vi "LabVIEW MakerHub Speed Direction State Machine.vi"() -> ()   [LabVIEW 2011]
panel:
  out "Speed Chart":dbl(graph)
  in  "Idle":bool
  out "State":T1(ring)=enum."fullreverse"
  in  "Max Speed":dbl=1.0
  in  "Acceleration":dbl=0.001
  in  "Stop Button":bool
  in  "Reverse":bool
  in  "Forward":bool
  out "Direction":bool
  out "Speed":dbl(knob)=1.0 scale=0.0..1.0
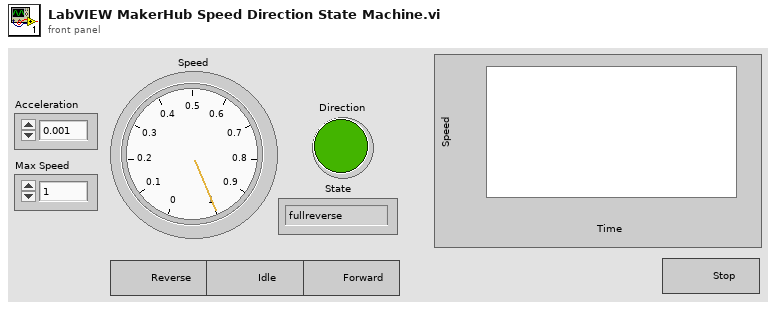
[diagram p1: front panel]
types:
  T1 = enum16{"idle", "accelerate", "fullforward", "decelerate", "fullreverse", "stop"}
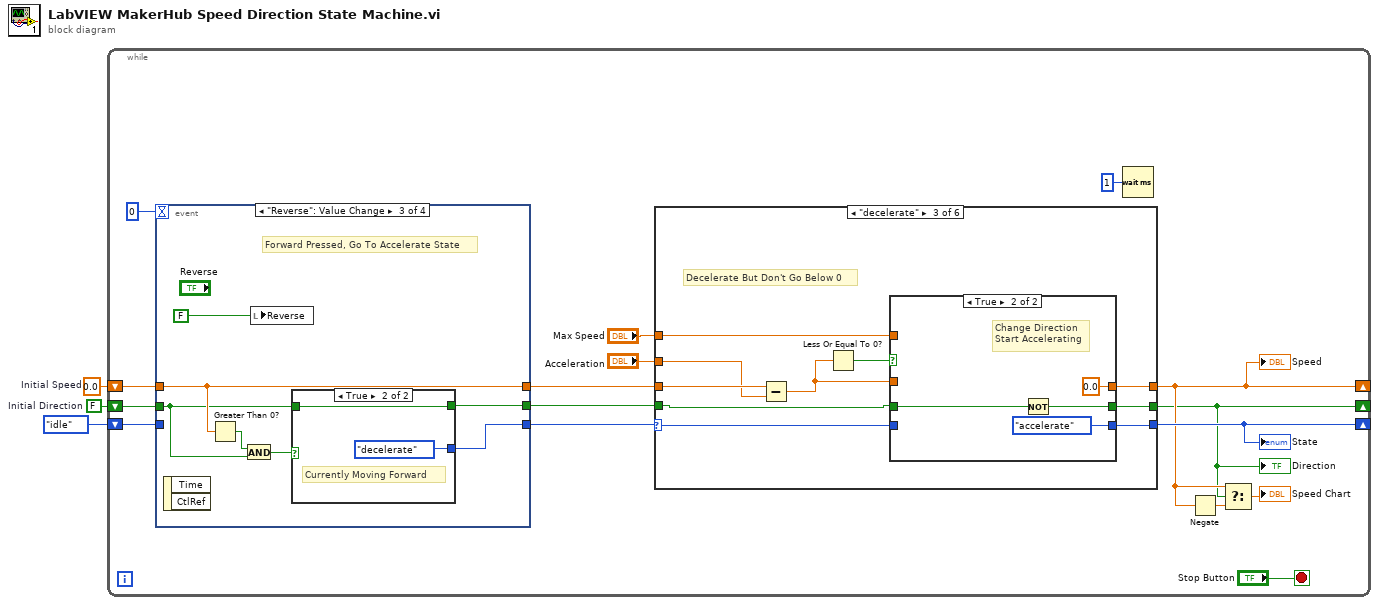
[diagram p0: block diagram]
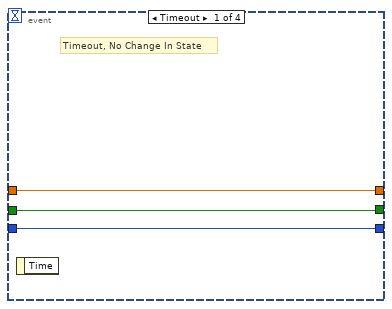
[diagram p2: hidden frame]
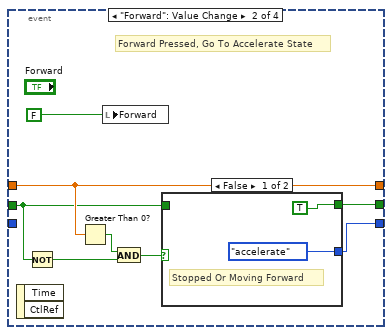
[diagram p3: hidden frame]
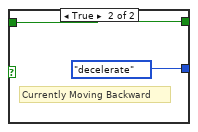
[diagram p4: hidden frame]
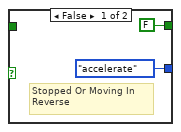
[diagram p5: hidden frame]
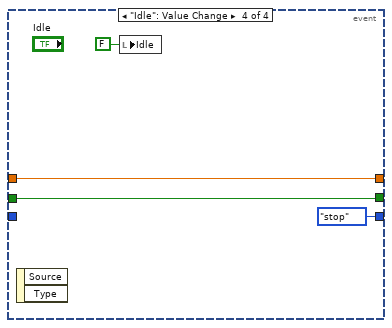
[diagram p6: hidden frame]
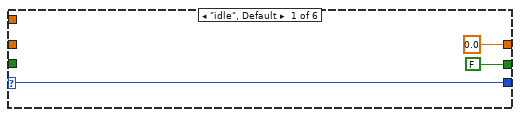
[diagram p7: hidden frame]
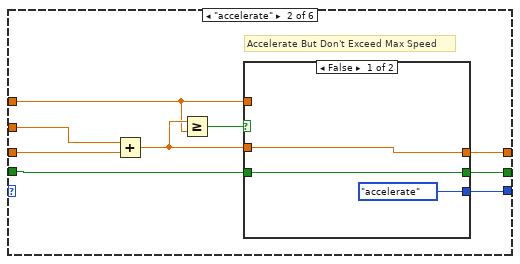
[diagram p8: hidden frame]
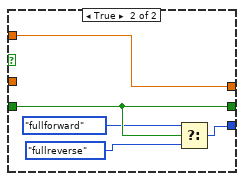
[diagram p9: hidden frame]
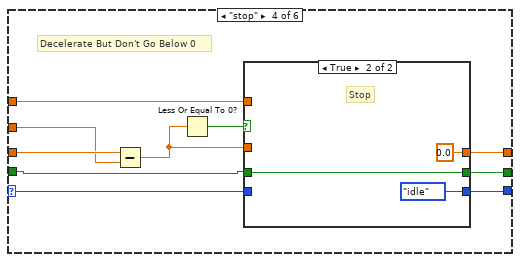
[diagram p11: hidden frame]
diagram:
  w1 = FALSE  # Initial Direction
  w2 = 0.0  # Initial Speed
  n1 = while {
    shift-right: [w6] -> _
    shift-left: w2 -> [w15]
    shift-right: [w12] -> _
    shift-left: T1."idle" -> [w18]
    shift-right: [w5] -> _
    shift-left: w1 -> [w13]
    stop <- "Stop Button" stop-if-true
    n2 = event shown="[2] \"Reverse\": Value Change" {
      selector: _ -> [_ _ _ _]
      dyn-events: _ -> [_ _ _ _]
      timeout: 0 -> [_ _ _ _]
      tunnel: [w22 w25 w39 T1."stop"] -> w17
      tunnel: w18 -> [w22 _ _ _]
      tunnel: [w21 w29 w40 w47] -> w16
      tunnel: w15 -> [w21 w29 w40 w47]
      tunnel: [w20 w23 w38 w46] -> w14
      tunnel: w13 -> [w20 w24 w36 w46]
      event Timeout {
        # "Timeout, No Change In State"
        n3 = event-data() -> ()  [unwired: 1 in, 1 out]
      }
      event "Forward": Value Change {
        # "Forward Pressed, Go To Accelerate State"
        n4 = event-data() -> ()  [unwired: 1 in, 2 out]
        n5 = Not(x=w24) -> (.not. x?=w27:bool)
        n6 = Greater Than 0?(x=w29) -> (x > 0?=w28:bool)
        n7 = local write "Forward"(FALSE ("Seek Back Button")) -> ()
        n8 = And(x=w28, y=w27) -> (x .and. y?=w26:bool)
        n9 = case shown="False" w26 {
          tunnel: [T1."accelerate" T1."decelerate"] -> w25
          tunnel: [TRUE ("Initial Direction") w33] -> w23
          tunnel: w24 -> [_ w33]
          frame False {
            # "Stopped Or Moving Forward"
          }
          frame True {
            # "Currently Moving Backward"
          }
        }
      }
      event "Reverse": Value Change {
        # "Forward Pressed, Go To Accelerate State"
        n10 = event-data() -> ()  [unwired: 1 in, 2 out]
        n11 = Greater Than 0?(x=w40) -> (x > 0?=w37:bool)
        n12 = And(x=w37, y=w36) -> (x .and. y?=w35:bool)
        n13 = local write "Reverse"(FALSE ("Seek Back Button")) -> ()
        n14 = case shown="True" w35 {
          tunnel: [T1."accelerate" T1."decelerate"] -> w39
          tunnel: [FALSE ("Initial Direction") w44] -> w38
          tunnel: w36 -> [_ w44]
          frame False {
            # "Stopped Or Moving In \nReverse"
          }
          frame True {
            # "Currently Moving Forward"
          }
        }
      }
      event "Idle": Value Change {
        n15 = event-data() -> ()  [unwired: 1 in, 2 out]
        n16 = local write "Idle"(FALSE ("Idle")) -> ()
      }
    }
    n17 = case shown="\"decelerate\"" w17 {
      selector: w17 -> [w50 _ w70 w87 w103 w106]
      tunnel: w16 -> [_ w61 w79 w96 w105 w108]
      tunnel: w14 -> [_ w55 w73 w90 w104 w107]
      tunnel: [0.0 ("Initial Speed") w58 w76 w93 w105 w108] -> w6
      tunnel: [FALSE ("Initial Direction") w54 w72 w89 w104 w107] -> w5
      tunnel: [w50 w56 w74 w91 w103 w106] -> w12
      tunnel: "Acceleration" -> [_ w60 w78 w95 _ _]
      tunnel: "Max Speed" -> [_ w53 w71 w88 _ _]
      frame "idle", Default {
      }
      frame "accelerate" {
        # "Accelerate But Don't Exceed Max Speed"
        n18 = Add(x=w60, y=w61) -> (x+y=w57:dbl)
        n19 = Greater Or Equal?(x=w57, y=w53) -> (x >= y?=w59:bool)
        n20 = case shown="False" w59 {
          tunnel: [w64 w69] -> w58
          tunnel: w53 -> [_ w69]
          tunnel: w57 -> [w64 _]
          tunnel: [T1."accelerate" w66] -> w56
          tunnel: w55 -> [w62 w68]
          tunnel: [w62 w68] -> w54
          frame False {
          }
          frame True {
            n21 = Select(t=T1."fullforward", s=w68, f=T1."fullreverse") -> (s? t:f=w66:T1)
          }
        }
      }
      frame "decelerate" {
        # "Decelerate But Don't Go Below 0"
        n22 = Subtract(x=w79, y=w78) -> (x-y=w75:dbl)
        n23 = Less Or Equal To 0?(x=w75) -> (x <= 0?=w77:bool)
        n24 = case shown="True" w77 {
          tunnel: [w82 0.0] -> w76
          tunnel: w71 -> [_ _]
          tunnel: w75 -> [w82 _]
          tunnel: [w80 T1."accelerate"] -> w74
          tunnel: w73 -> [w81 w84]
          tunnel: [w81 w83] -> w72
          tunnel: w70 -> [w80 _]
          frame False {
          }
          frame True {
            # "Change Direction\nStart Accelerating"
            n25 = Not(x=w84) -> (.not. x?=w83:bool)
          }
        }
      }
      frame "stop" {
        # "Decelerate But Don't Go Below 0"
        n26 = Subtract(x=w96, y=w95) -> (x-y=w92:dbl)
        n27 = Less Or Equal To 0?(x=w92) -> (x <= 0?=w94:bool)
        n28 = case shown="True" w94 {
          tunnel: [w99 0.0] -> w93
          tunnel: w88 -> [_ _]
          tunnel: w92 -> [w99 _]
          tunnel: [w97 T1."idle"] -> w91
          tunnel: w90 -> [w98 w100]
          tunnel: [w98 w100] -> w89
          tunnel: w87 -> [w97 _]
          frame False {
          }
          frame True {
            # "Stop"
          }
        }
      }
      frame "fullforward" {
      }
      frame "fullreverse" {
      }
    }
    "Speed" <- w6
    "Direction" <- w5
    "State" <- w12
    n29 = Wait (ms)(milliseconds to wait=u32 1) -> ()  [unwired: 1 out]
    n30 = Negate(x=w6) -> (-x=w7:dbl)
    n31 = Select(t=w6, s=w5, f=w7) -> (s? t:f=→"Speed Chart":dbl)
  }
